vi "IsCarInFront.vi"(1 "Sensor Links":dbl, 2 "Sensor Rechts":dbl) -> (0 "IsFollowingAuto":bool)   [LabVIEW 2016]
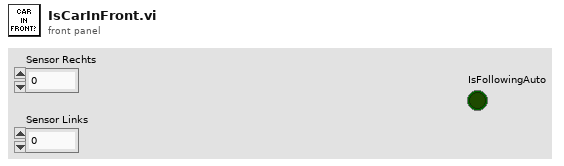
[diagram p1: front panel]
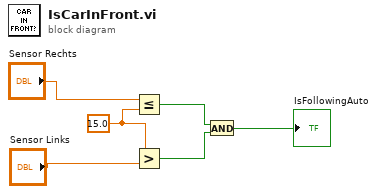
[diagram p0: block diagram]
diagram:
  w5 = 15.0 ("y")
  n1 = Less Or Equal?(x="Sensor Rechts", y=w5) -> (x <= y?=w3:bool)
  n2 = Greater?(x=w5, y="Sensor Links") -> (0:w2:bool)
  n3 = And(x=w3, y=w2) -> (x .and. y?=→"IsFollowingAuto":bool)
